vi "tm_getemprotectstatus_40.vi"(8 "error in (no error)":errorcluster {"code" format="%.0x"}, 11 "Handle in":u32) -> (0 "error out":errorcluster {"code" format="%.0x"}, 2 "Status":i32, 3 "Handle out":u32)   [LabVIEW 2011]
uses:
  tmcamcon.dll
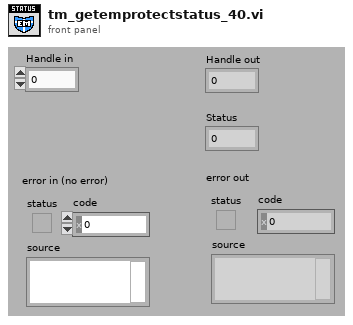
[diagram p1: front panel]
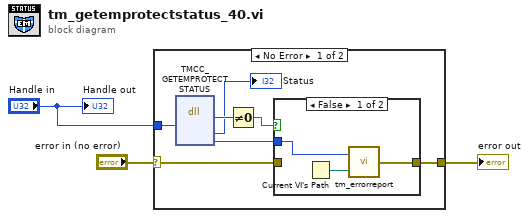
[diagram p0: block diagram]
diagram:
  n1 = case shown="No Error" "error in (no error)" {
    selector: "error in (no error)" -> [w10 w15]
    tunnel: [w8 w15] -> w1
    tunnel: "Handle in" -> [w5 _]
    frame No Error {
      n2 = dll-call lib="tmcamcon.dll" fn="TMCC_GETEMPROTECTSTATUS"("index"=w5) -> ("return type"=w7:u32, "status"=→"Status":i32, "Erval"=w6:i32)  [unwired: 6 in, 2 out]
      n3 = Not Equal To 0?(x=w7) -> (x != 0?=w9:bool)
      n4 = case shown="False" w9 {
        tunnel: w10 -> [_ w14]
        tunnel: [w11 w14] -> w8
        tunnel: w6 -> [w12 _]
        frame False {
          n5 = Current VI's Path() -> (path=w13:path)
          n6 = call <userlib>:"tm_errorreport.vi"("Source"=w13, "Error"=w12) -> ("error out"=w11:errorcluster)
        }
        frame True {
        }
      }
    }
    frame Error {
    }
  }
  "error out" <- w1
  "Handle out" <- "Handle in"
